vi "FlushSerial.vi"(8 "error in":errorcluster, 11 "Python":T1) -> (0 "error out":errorcluster, 3 "Python":T1)   [LabVIEW 2022 SP3]
uses:
  PythonCtrl.ctl
  Processors.ctl
panel:
  out "return value":i32
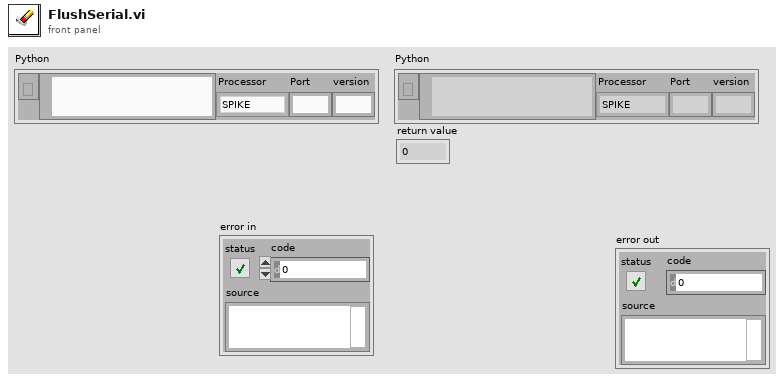
[diagram p1: front panel]
types:
  T1 = typedef "PythonCtrl.ctl" = cluster{"session":refnum<k35>, "PyPath":path, "Processor":T2, "Port":string, "version":string}
  T2 = typedef "Processors.ctl" = enum16{"SPIKE", "Pi", "Pi_ssh", "OpenMV", "Dunio"}
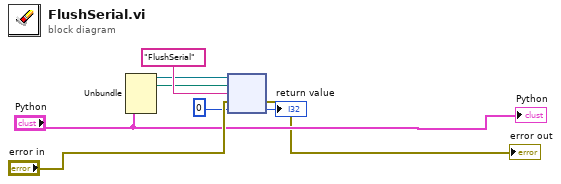
[diagram p0: block diagram]
diagram:
  n1 = Unbundle("Python") -> ("session"=w4:refnum<k35>, "PyPath"=w3:path)  [unwired: 3 out]
  n2 = node(w4, w3, "FlushSerial" ("function name"), "error in", 0 ("function name")) -> (→"error out":errorcluster, →"return value":i32)  [unwired: 3 out]
  "Python" <- "Python"
